vi "UserVars-Substitute Constants.vi"(7 "Expression In":string) -> (8 "Expression Out":string)   [LabVIEW 2020]
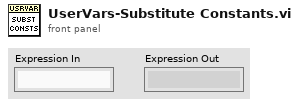
[diagram p1: front panel]
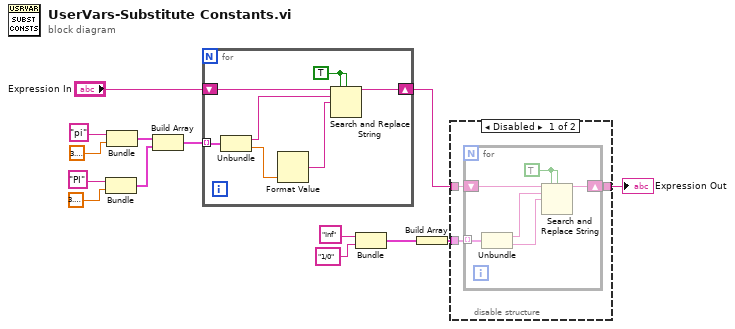
[diagram p0: block diagram]
diagram:
  n1 = Bundle("PI", 3.141592653589793) -> (w2:cluster{string, dbl})  [unwired: 1 in]
  n2 = Bundle("pi", 3.141592653589793) -> (w12:cluster{string, dbl})  [unwired: 1 in]
  n3 = Build Array(w12, w2) -> (w10:cluster{string, dbl}[])
  n4 = for {
    shift-right: [w18] -> w7
    shift-left: "Expression In" -> [w19]
    tunnel: w10 -> [w21] mode=indexing
    w17 = TRUE ("replace all? (F)")
    n5 = Unbundle(w21) -> (w16:string, w20:dbl)
    n6 = Format Value(value (0)=w20) -> (output string=w15:string)  [unwired: 2 in]
    n7 = Search and Replace String(replace all?=w17, case sensitive?=w17, input string=w19, search string=w16, replace string=w15) -> (result string=w18:string)  [unwired: 3 in, 3 out]
  }
  n8 = Bundle("Inf", "1/0") -> (w6:cluster{string, string})  [unwired: 1 in]
  n9 = Build Array(w6) -> (w1:cluster{string, string}[])
  n10 = disable-structure shown="Disabled" {
    disable-tunnel: w7 -> [w24 w31]
    disable-tunnel: [w23 w31] -> w5
    disable-tunnel: w1 -> [w22 _]
    frame Disabled {
      n11 = for {
        shift-right: [w28] -> w23
        shift-left: w24 -> [w29]
        tunnel: w22 -> [w30] mode=indexing
        w27 = TRUE ("replace all? (F)")
        n12 = Unbundle(w30) -> (w26:string, w25:string)
        n13 = Search and Replace String(replace all?=w27, case sensitive?=w27, input string=w29, search string=w26, replace string=w25) -> (result string=w28:string)  [unwired: 3 in, 3 out]
      }
    }
    frame Enabled {
    }
  }
  "Expression Out" <- w5
